vi "niRFUtil CONV 1 Ohm Voltage to 1 Ohm Watt (complex array).vi"(7 "Complex Array (V)":T2 format="%.2f") -> (8 "Real Array (W)":T1 min=0 max=127 format="%.2f")   [LabVIEW 2015, in "niRFUtil.lvlib"]
doc: "(c) Copyright 2006, National Instruments, Inc. This VI may not be duplicated, sold, or distributed without written consent from National Instruments."
uses:
  niRFUtil.lvlib
  Includes/niRFUtil INC Complex Array.ctl
  Includes/niRFUtil INC Real Array.ctl
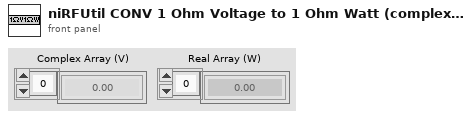
[diagram p1: front panel]
types:
  T1 = typedef "niRFUtil.lvlib/niRFUtil INC Real Array.ctl" = sgl[]
  T2 = typedef "niRFUtil.lvlib/niRFUtil INC Complex Array.ctl" = csg[]
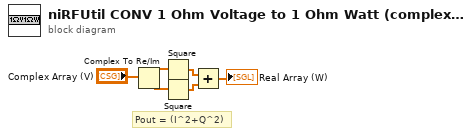
[diagram p0: block diagram]
diagram:
  # "Pout = (I^2+Q^2)"
  n1 = Complex To Re/Im(x + iy="Complex Array (V)") -> (x=w6:sgl[], y=w5:sgl[])
  n2 = Square(x=w6) -> (x^2=w4:sgl[])
  n3 = Square(x=w5) -> (x^2=w3:sgl[])
  n4 = Add(x=w4, y=w3) -> (x+y=→"Real Array (W)":sgl[])
